vi "acquisitionGetZLatestVolume.vi"(1 "nFramesLatestVolume":i32, 2 "firstFrameCountLatestVolume":i32) -> (0 "z latest volume":dbl[](array[numeric]))   [LabVIEW 2017]
uses:
  globalDevices.vi
  globalUtilities.vi
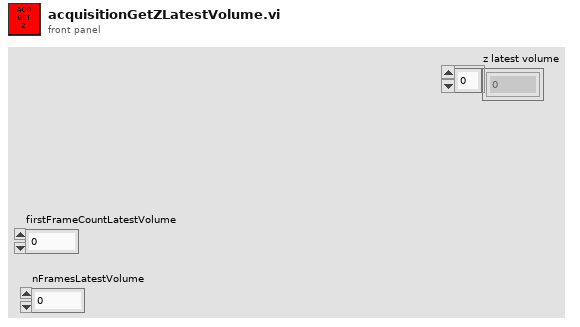
[diagram p1: front panel]
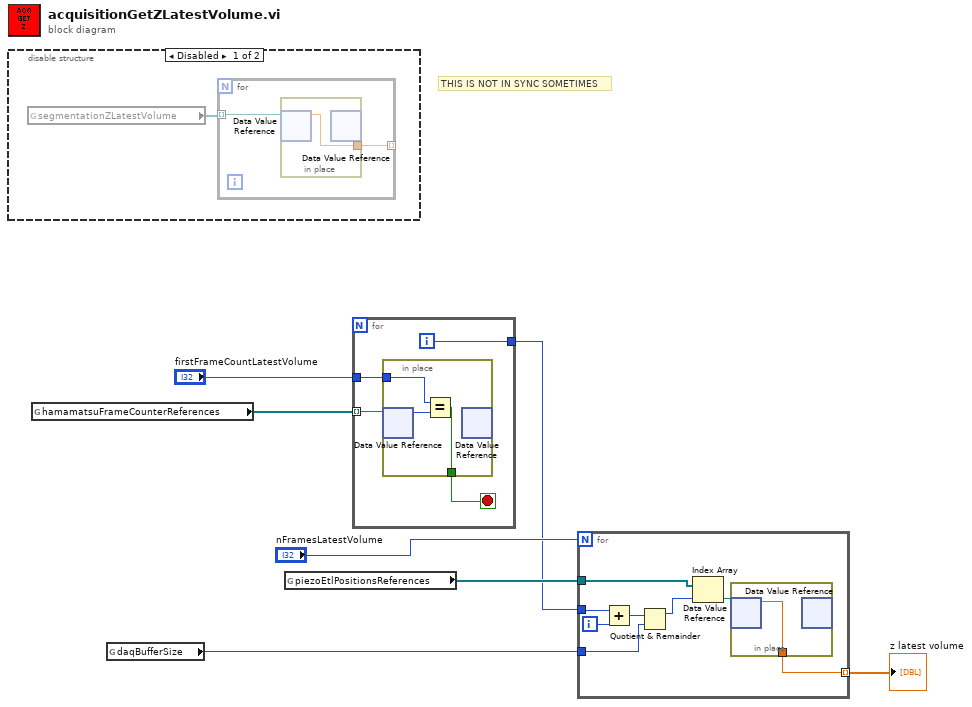
[diagram p0: block diagram]
diagram:
  # "THIS IS NOT IN SYNC SOMETIMES"
  n1 = disable-structure shown="Disabled" {
    frame Disabled {
      n2 = global read "globalUtilities.vi" "segmentationZLatestVolume"() -> (w8:refnum<data-value>[])
      n3 = for {
        tunnel: w8 -> [w10] mode=indexing
        tunnel: [w9] -> _ mode=indexing
        n4 = in-place {
          in-place-border: [w11] -> w9
          n5 = in-place-dvr #1(w10) -> (w11:dbl)  [unwired: 1 out]
          n6 = in-place-dvr #1() -> ()  [unwired: 1 in, 2 out]
        }
      }
    }
    frame Enabled {
    }
  }
  n7 = global read "globalDevices.vi" "hamamatsuFrameCounterReferences"() -> (w7:refnum<data-value>[])
  n8 = global read "globalDevices.vi" "daqBufferSize"() -> (w2:i32)
  n9 = global read "globalDevices.vi" "piezoEtlPositionsReferences"() -> (w5:refnum<data-value>[])
  n10 = for {
    tunnel: w7 -> [w15] mode=indexing
    tunnel: "firstFrameCountLatestVolume" -> [w14]
    tunnel: [w12] -> w3
    i -> [w12]
    stop <- w13 stop-if-true
    n11 = in-place {
      in-place-border: w14 -> [w17]
      in-place-border: [w16] -> w13
      n12 = in-place-dvr #2(w15) -> (w18:u32)  [unwired: 1 out]
      n13 = Equal?(x=w17, y=w18) -> (x = y?=w16:bool)
      n14 = in-place-dvr #2() -> ()  [unwired: 1 in, 2 out]
    }
  }
  n15 = for {
    N: "nFramesLatestVolume" -> [_]
    tunnel: w5 -> [w22]
    tunnel: w3 -> [w26]
    tunnel: w2 -> [w23]
    tunnel: [w19] -> w1 mode=indexing
    i -> [w25]
    n16 = Add(x=w26, y=w25) -> (x+y=w24:i32)
    n17 = Quotient & Remainder(x=w24, y=w23) -> (x-y*floor(x/y)=w21:i32)  [unwired: 1 out]
    n18 = Index Array(array=w22, index=w21) -> (element=w20:refnum<data-value>)
    n19 = in-place {
      in-place-border: [w27] -> w19
      n20 = in-place-dvr #3(w20) -> (w27:dbl)  [unwired: 1 out]
      n21 = in-place-dvr #3() -> ()  [unwired: 1 in, 2 out]
    }
  }
  "z latest volume" <- w1
